vi "Main.vi"() -> ()   [LabVIEW 2015]
uses:
  TypDefs/Loop States.ctl
  TypDefs/Loop Data.ctl
panel:
  in  "device name":tag="myDAQ1"
  in  "Exit Button":bool
  in  "Start Button":bool
  out "Status":string
  in  "Clear Button":bool
  in  "Save Button":bool
  out "XY Graph":cluster{"X":dbl[], "Y":dbl[]}(graph)
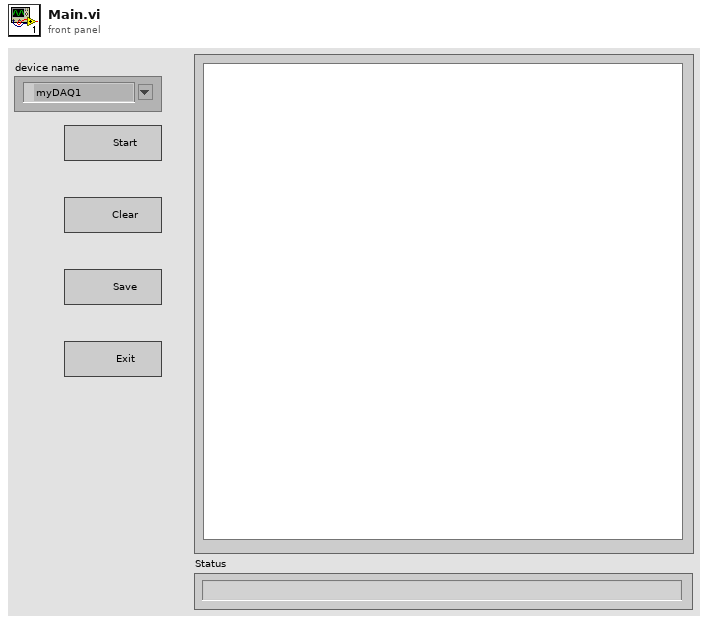
[diagram p1: front panel]
types:
  T1 = typedef "Loop Data.ctl" = cluster{"Status":string, "Graph Data":cluster{"X":dbl[], "Y":dbl[]}, "Recording Status":bool}
  T2 = typedef "Loop States.ctl" = enum16{"Error", "Wait for events", "Measure positions", "Update UI", "Initialization"}
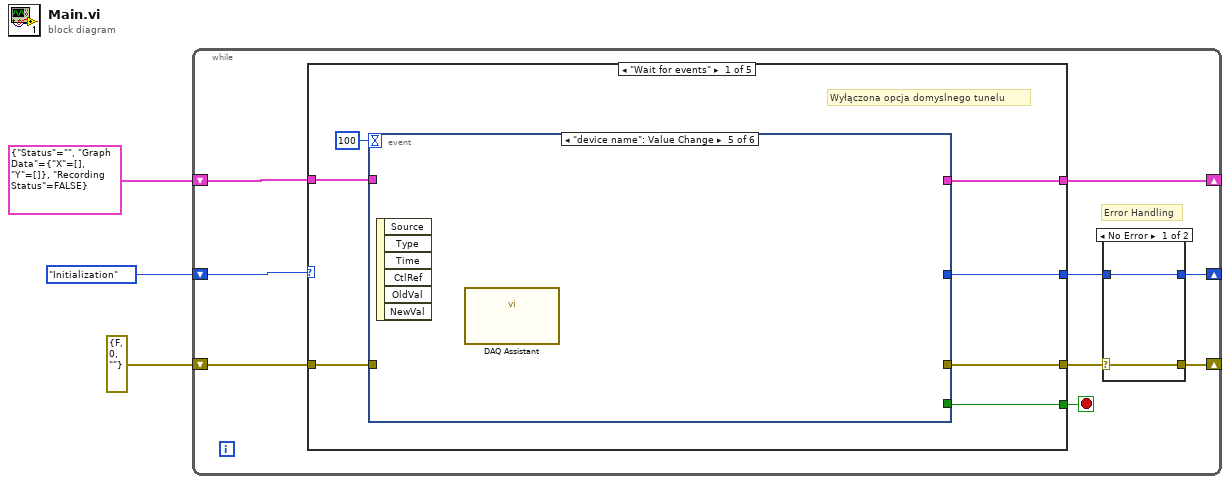
[diagram p0: block diagram]
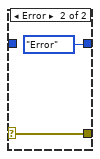
[diagram p2: hidden frame]
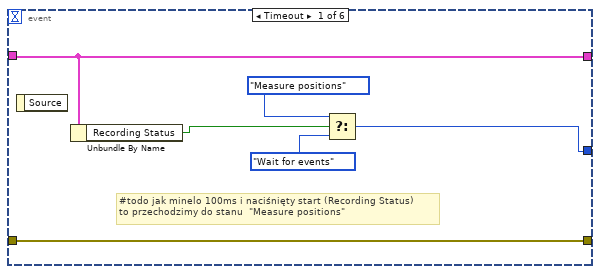
[diagram p3: hidden frame]
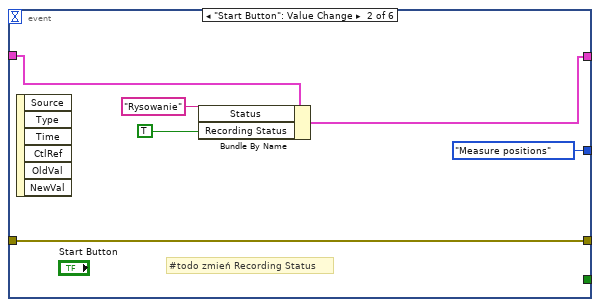
[diagram p4: hidden frame]
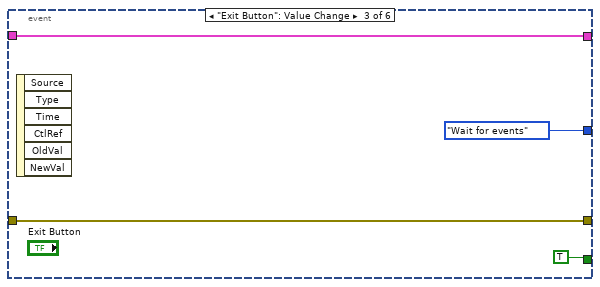
[diagram p5: hidden frame]
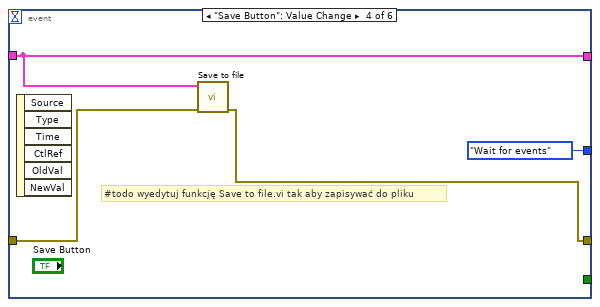
[diagram p6: hidden frame]
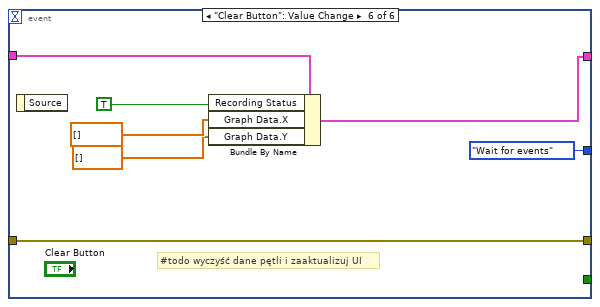
[diagram p7: hidden frame]
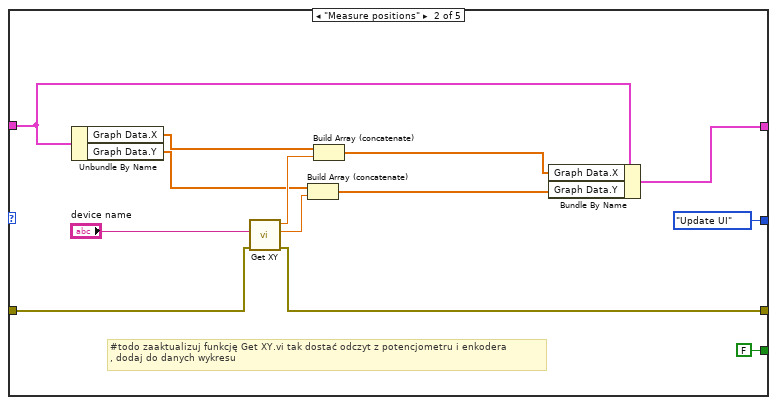
[diagram p8: hidden frame]
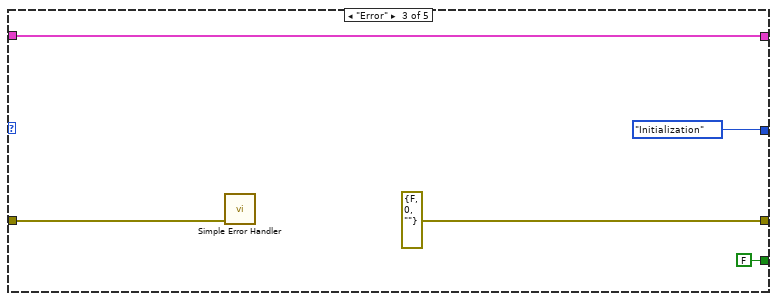
[diagram p9: hidden frame]
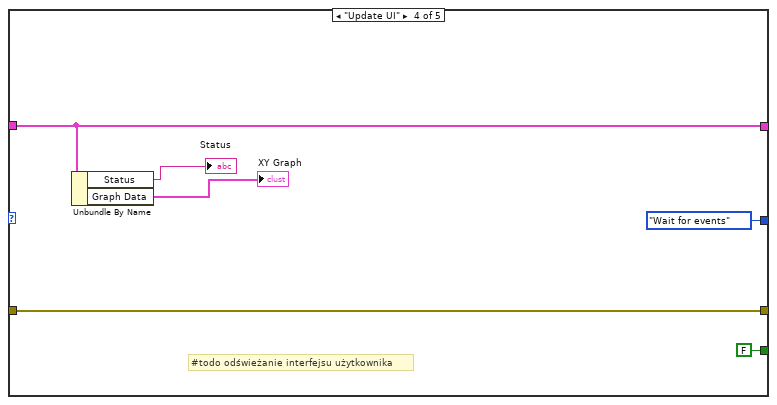
[diagram p10: hidden frame]
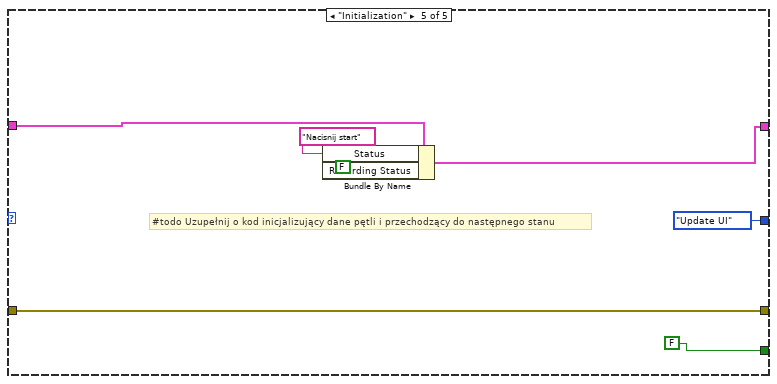
[diagram p11: hidden frame]
diagram:
  n1 = while {
    shift-right: [w10] -> _
    shift-left: T1 {"Status"="", "Graph Data"={"X"=[], "Y"=[]}, "Recording Status"=FALSE} -> [w11]
    shift-right: [w5] -> _
    shift-left: Loop_States."Initialization" -> [w12]
    shift-right: [w4] -> _
    shift-left: errorcluster {"status"=FALSE, "code"=0, "source"=""} ("error constant") -> [w8]
    stop <- w9 stop-if-true
    # "Error Handling"
    n2 = case shown="\"Wait for events\"" w12 {
      tunnel: w11 -> [w22 w61 w65 w71 w79]
      tunnel: [w20 w63 w65 w71 w78] -> w10
      tunnel: [w19 FALSE FALSE FALSE FALSE] -> w9
      tunnel: [w21 Loop_States."Update UI" Loop_States."Initialization" Loop_States."Wait for events" Loop_States."Update UI"] -> w6
      tunnel: w8 -> [w18 w53 w67 w73 w76]
      tunnel: [w17 w54 errorcluster {"status"=FALSE, "code"=0, "source"=""} ("error constant") w73 w76] -> w7
      frame "Wait for events" {
        # "Wyłączona opcja domyslnego tunelu"
        n3 = event shown="[4] \"device name\": Value Change" {
          selector: _ -> [_ _ _ _ _ _]
          dyn-events: _ -> [_ _ _ _ _ _]
          timeout: 100 -> [_ _ _ _ _ _]
          tunnel: w22 -> [w28 w35 w38 w40 _ w49]
          tunnel: [w26 Loop_States."Measure positions" Loop_States."Wait for events" Loop_States."Wait for events" _ Loop_States."Wait for events"] -> w21
          tunnel: [w28 w32 w38 w40 _ w44] -> w20
          tunnel: [_ _ TRUE _ _ _] -> w19
          tunnel: w18 -> [w29 w31 w36 w42 _ w45]
          tunnel: [w29 w31 w36 w41 _ w45] -> w17
          event Timeout {
            # "#todo jak minelo 100ms i naciśnięty start (Recording Status) \nto przechodzimy do stanu  \"Measure positions\""
            n4 = event-data() -> ()  [unwired: 1 in, 1 out]
            n5 = Unbundle By Name(w28) -> ("Recording Status"=w27:bool)
            n6 = Select(t=Loop_States."Measure positions", s=w27, f=Loop_States."Wait for events") -> (s? t:f=w26:T2)
          }
          event "Start Button": Value Change {
            # "#todo zmień Recording Status"
            n7 = event-data() -> ()  [unwired: 1 in, 6 out]
            n8 = Bundle By Name(cluster=w35, "Status"="Rysowanie", "Recording Status"=TRUE) -> (w32:T1)
          }
          event "Exit Button": Value Change {
            n9 = event-data() -> ()  [unwired: 1 in, 6 out]
          }
          event "Save Button": Value Change {
            # "#todo wyedytuj funkcję Save to file.vi tak aby zapisywać do pliku"
            n10 = event-data() -> ()  [unwired: 1 in, 6 out]
            n11 = call "Save to file.vi"("error in (no error)"=w42, "Loop Data"=w40) -> ("error out"=w41:errorcluster)  [unwired: 9 in]
          }
          event "device name": Value Change {
            n12 = event-data() -> ()  [unwired: 1 in, 6 out]
            n13 = call "DAQ Assistant"() -> ()  [unwired: 12 in]
          }
          event "Clear Button": Value Change {
            # "#todo wyczyść dane pętli i zaaktualizuj UI"
            n14 = event-data() -> ()  [unwired: 1 in, 1 out]
            n15 = Bundle By Name(cluster=w49, "Recording Status"=TRUE, "Graph Data.X"=dbl[] [], "Graph Data.Y"=dbl[] []) -> (w44:T1)
          }
        }
      }
      frame "Measure positions" {
        # "#todo zaaktualizuj funkcję Get XY.vi tak dostać odczyt z potencjometru i enkodera \n, dodaj do danych wykresu"
        n16 = Unbundle By Name(w61) -> ("Graph Data.X"=w59:dbl[], "Graph Data.Y"=w56:dbl[])
        n17 = call "Get XY.vi"("error in"=w53, "device name"="device name") -> ("error out"=w54:errorcluster, "Y"=w55:dbl, "X"=w58:dbl)  [unwired: 7 in]
        n18 = Build Array (concatenate)(w56, w55) -> (w52:dbl[])
        n19 = Build Array (concatenate)(w59, w58) -> (w57:dbl[])
        n20 = Bundle By Name(cluster=w61, "Graph Data.X"=w57, "Graph Data.Y"=w52) -> (w63:T1)
      }
      frame "Error" {
        n21 = call <vilib>:"Simple Error Handler.vi"("error in (no error)"=w67) -> ()  [unwired: 4 in, 5 out]
      }
      frame "Update UI" {
        # "#todo odświeżanie interfejsu użytkownika"
        n22 = Unbundle By Name(w71) -> ("Status"=→"Status":string, "Graph Data"=→"XY Graph":cluster{"X":dbl[], "Y":dbl[]})
      }
      frame "Initialization" {
        # "#todo Uzupełnij o kod inicjalizujący dane pętli i przechodzący do następnego stanu"
        n23 = Bundle By Name(cluster=w79, "Status"="Nacisnij start", "Recording Status"=FALSE) -> (w78:T1)
      }
    }
    n24 = case shown="No Error" w7 {
      selector: w7 -> [w13 w15]
      tunnel: w6 -> [w14 _]
      tunnel: [w14 Loop_States."Error"] -> w5
      tunnel: [w13 w15] -> w4
      frame No Error {
      }
      frame Error {
      }
    }
  }
